vi "INDEX-format-input.vi"(10 "tasks":T2[](array[typedef])) -> (1 "HTML":string[](array[string]), 2 "states":T1[](array[typedef]))   [LabVIEW 2014]
uses:
  controls/state program.ctl
  controls/state-machine.ctl
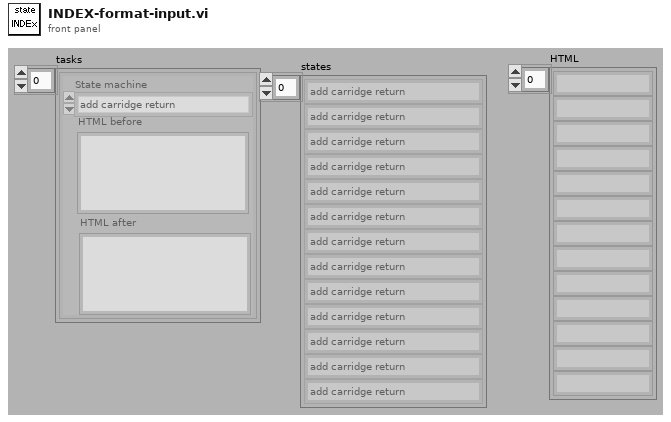
[diagram p1: front panel]
types:
  T1 = typedef "state-machine.ctl" = enum16{"add carridge return", "init", "Read-inputs", "edit generated file", "end", "Add front panel", "Add Block Diagram", "Add VI icon", "Add VI description", "Add VI hiearchy", "Add list of sub vis", "add custom html", "open report in browser", "Save report to file", "dispose report", "Add header text", "Create style .css", "add-red-box-header", "Delete Temp Files", "Remove-path-element", "add-revision-history", "add-icon-image-only"}
  T2 = typedef "state program.ctl" = cluster{"State machine":T1, "HTML before":string, "HTML after":string}
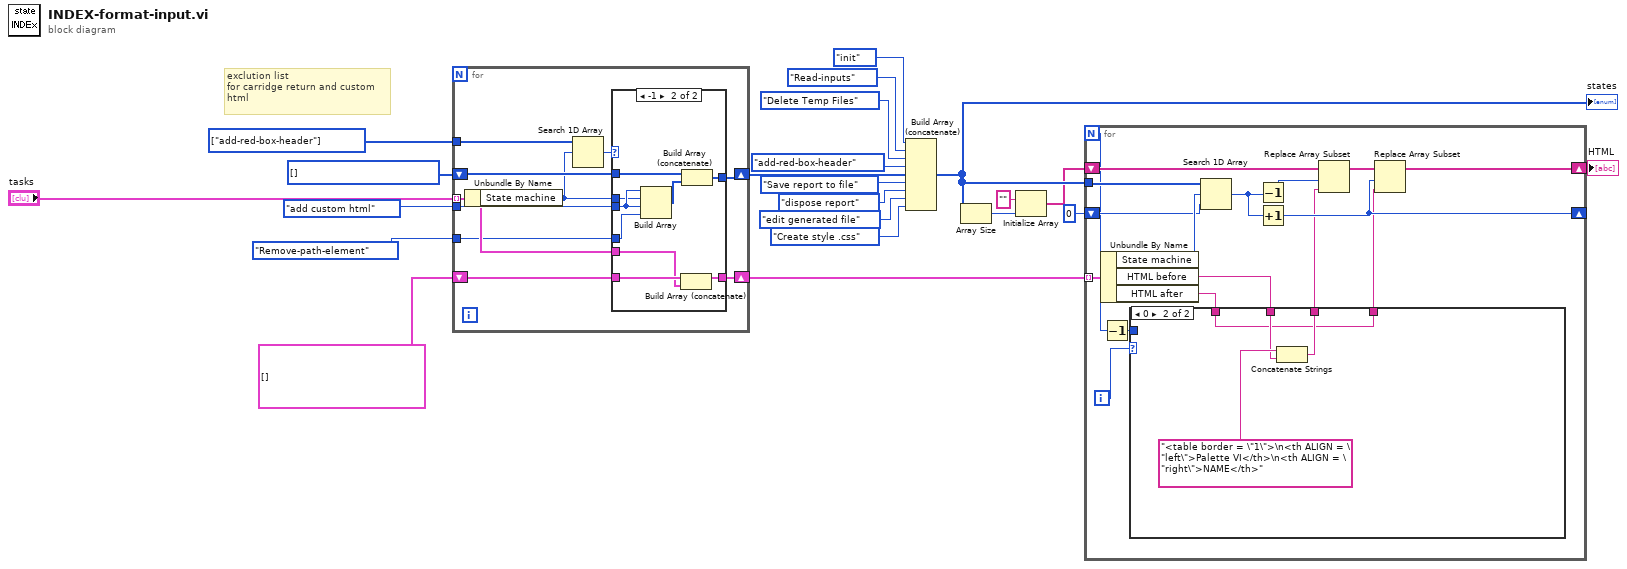
[diagram p0: block diagram]
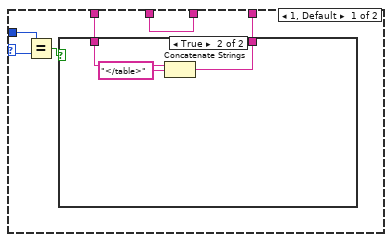
[diagram p2: hidden frame]
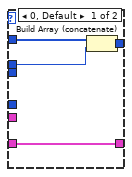
[diagram p4: hidden frame]
diagram:
  w22 = T1[] [enum."add-red-box-header"] items=["add carridge return", "init", "Read-inputs", "edit generated file", "end", "Add front panel", "Add Block Diagram", "Add VI icon", "Add VI description", "Add VI hiearchy", "Add list of sub vis", "add custom html", "open report in browser", "Save report to file", "dispose report", "Add header text", "Create style .css", "add-red-box-header", "Delete Temp Files", "Remove-path-element", "add-revision-history", "add-icon-image-only"]
  w8 = T1[] [] items=["add carridge return", "init", "Read-inputs", "edit generated file", "end", "Add front panel", "Add Block Diagram", "Add VI icon", "Add VI description", "Add VI hiearchy", "Add list of sub vis", "add custom html", "open report in browser", "Save report to file", "dispose report", "Add header text", "Create style .css", "add-red-box-header", "Delete Temp Files", "Remove-path-element", "add-revision-history", "add-icon-image-only"]
  # "exclution list\nfor carridge return and custom\nhtml"
  n1 = for {
    tunnel: "tasks" -> [w24] mode=indexing
    tunnel: state-machine."add custom html" ("State machine") -> [w30]
    shift-right: [w31] -> w17
    shift-left: w8 -> [w32]
    tunnel: w22 -> [w27]
    shift-right: [w26] -> w7
    shift-left: T2[] [] -> [w25]
    tunnel: state-machine."Remove-path-element" ("State machine") -> [w23]
    n2 = Unbundle By Name(w24) -> ("State machine"=w29:T1)
    n3 = Search 1D Array(1D array=w27, element=w29) -> (index of element=w28:i32)  [unwired: 1 out]
    n4 = case shown="-1" w28 {
      tunnel: w32 -> [w36 w44]
      tunnel: [w35 w43] -> w31
      tunnel: w29 -> [w34 w41]
      tunnel: w30 -> [_ w42]
      tunnel: [w33 w40] -> w26
      tunnel: w25 -> [w33 w39]
      tunnel: w24 -> [_ w38]
      tunnel: w23 -> [_ w37]
      frame 0, Default {
        n5 = Build Array (concatenate)(w36, w34) -> (w35:T1[])
      }
      frame -1 {
        n6 = Build Array(w42, w41, w42, w37) -> (w45:T1[])
        n7 = Build Array (concatenate)(w39, w38) -> (w40:T2[])
        n8 = Build Array (concatenate)(w44, w45) -> (w43:T1[])
      }
    }
  }
  n9 = Build Array (concatenate)(state-machine."init" ("element"), state-machine."Read-inputs" ("element"), state-machine."Delete Temp Files" ("element"), state-machine."add-red-box-header" ("element"), w17, state-machine."Save report to file" ("element"), state-machine."dispose report" ("element"), state-machine."edit generated file" ("element"), state-machine."Create style .css" ("element")) -> (w12:T1[])
  "states" <- w12
  n10 = Array Size(array=w12) -> (size(s)=w11:i32)
  n11 = Initialize Array("", w11) -> (w9:string[])
  n12 = for {
    N -> [w49]
    tunnel: w12 -> [w62]
    tunnel: w7 -> [w61] mode=indexing
    shift-right: [w55] -> w5
    shift-left: w9 -> [w58]
    shift-right: [w54] -> _
    shift-left: 0 -> [w53]
    i -> [w50]
    n13 = Unbundle By Name(w61) -> ("State machine"=w60:T1, "HTML before"=w52:string, "HTML after"=w47:string)
    n14 = Decrement(x=w49) -> (x-1=w48:i32)
    n15 = case shown="0" w50 {
      selector: w50 -> [w67 _]
      tunnel: w52 -> [w68 w75]
      tunnel: [w68 w74] -> w51
      tunnel: w48 -> [w66 _]
      tunnel: w47 -> [w64 w73]
      tunnel: [w63 w73] -> w46
      frame 1, Default {
        n16 = Equal?(x=w66, y=w67) -> (x = y?=w65:bool)
        n17 = case shown="True" w65 {
          tunnel: w64 -> [w69 w72]
          tunnel: [w69 w71] -> w63
          frame False {
          }
          frame True {
            n18 = Concatenate Strings(w72, "</table>" ("string")) -> (w71:string)
          }
        }
      }
      frame 0 {
        n19 = Concatenate Strings("<table border = \"1\">\n<th ALIGN = \"left\">Palette VI</th>\n<th ALIGN = \"right\">NAME</th>", w75) -> (w74:string)
      }
    }
    n20 = Search 1D Array(1D array=w62, element=w60, start index (0)=w53) -> (index of element=w59:i32)
    n21 = Decrement(x=w59) -> (x-1=w56:i32)
    n22 = Increment(x=w59) -> (x+1=w54:i32)
    n23 = Replace Array Subset(array=w58, new element=w51, index=w56) -> (w57:string[])
    n24 = Replace Array Subset(array=w57, new element=w46, index=w54) -> (w55:string[])
  }
  "HTML" <- w5
